vi "write_amp_phase.vi"(8 "Index":i32, 9 "Phase (rad)":dbl, 10 "Amplitude (V)":dbl, 11 "Resonance Curve Data in":refnum<class "Resonance Curve Data.lvclass">) -> (3 "Resonance Curve Data out":refnum<class "Resonance Curve Data.lvclass">)   [LabVIEW 2020, in "Resonance Curve Data.lvclass"]
uses:
  Resonance Curve Data.lvclass
  Resonance Curve Data.lvclass/Resonance Curve Data.ctl
panel:
  # "Given a pair of amplitude and phase measurements, in-place update the resonance curve data at the specified index"
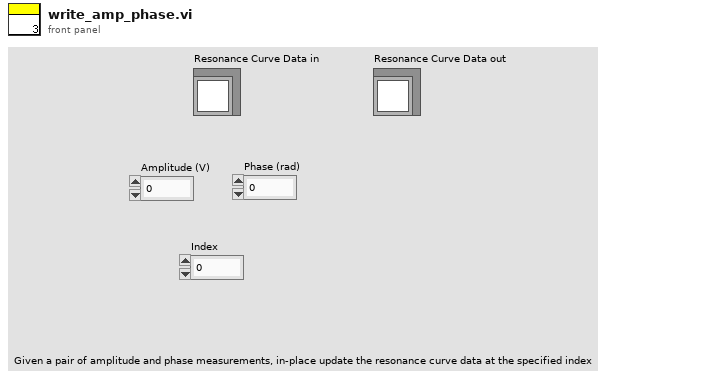
[diagram p1: front panel]
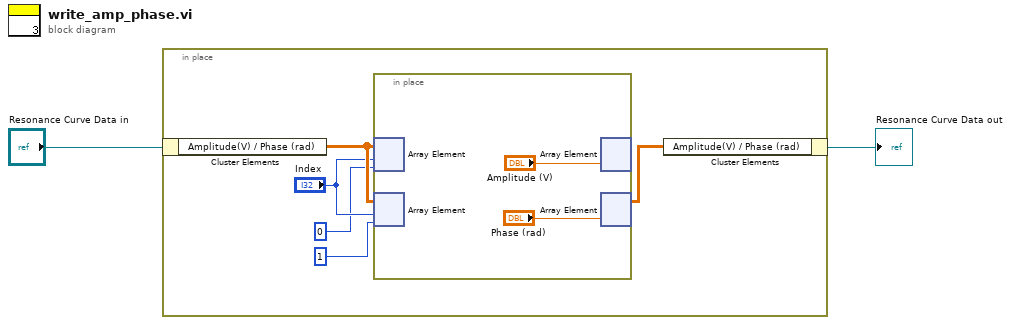
[diagram p0: block diagram]
diagram:
  n1 = in-place {
    n2 = in-place-cluster #1("Resonance Curve Data in") -> ("Amplitude(V) / Phase (rad)"=w7:dbl[][])
    n3 = in-place {
      n4 = in-place-array #2(w7, "Index", 0) -> ()  [unwired: 1 out]
      n5 = in-place-array #3(w7, "Index", 1) -> ()  [unwired: 1 out]
      n6 = in-place-array #2("Amplitude (V)") -> ()  [unwired: 3 out]
      n7 = in-place-array #3("Phase (rad)") -> (w3:dbl[][])  [unwired: 2 out]
    }
    n8 = in-place-cluster #1("Amplitude(V) / Phase (rad)"=w3) -> (→"Resonance Curve Data out":refnum<class "Resonance Curve Data.lvclass">)
  }
